vi "S4GUI.vi"() -> ()   [LabVIEW 2018] (continued)
            n2260 = call-dynamic "Write Observer.vi"("error in (no error)"=w5311, "Observer"=w5314, "Interface in"=w5310) -> ("error out"=w5306:errorcluster, "Interface out"=w5305:refnum<class "Interface.lvclass">)  [unwired: 7 in]
            n2261 = call-dynamic "Write Interface.vi"("error in (no error)"=w5306, "Interface.lvclass"=w5305, "Channel in"=w5325) -> ("error out"=w5301:errorcluster, "Channel out"=w5304:refnum<class "Channel.lvclass">)  [unwired: 7 in]
            n2262 = call-dynamic "Read State Machine.vi"("error in (no error)"=w5301, "Device in"=w5304) -> ("error out"=w5309:errorcluster, "State Machine.lvclass"=w5299:refnum<class "State Machine.lvclass">, "Device out"=w5303:refnum<class "Channel.lvclass">)  [unwired: 7 in]
            n2263 = call "Next State.vi"("error in (no error)"=w5309, "New_State"=12, "State Machine in"=w5299) -> ("error out"=w5308:errorcluster, "State Machine out"=w5298:refnum<class "State Machine.lvclass">)  [unwired: 7 in]
            n2264 = call-dynamic "Write State Machine.vi"("error in (no error)"=w5308, "State Machine.lvclass"=w5298, "Device in"=w5303) -> ("error out"=w5300:errorcluster, "Device out"=w5302:refnum<class "Channel.lvclass">)  [unwired: 7 in]
            n2265 = call-dynamic "Write Channel.vi"("error in (no error)"=w5300, "Channel.lvclass"=w5302, "Acquisition in"=w5320) -> ("error out"=w5318:errorcluster, "Acquisition out"=w5319:refnum<class "Acquisition.lvclass">)  [unwired: 7 in]
            n2266 = call-dynamic "Write AcquisitionD.vi"("error in (no error)"=w5318, "Acquisition.lvclass"=w5319, "S4ACS_GUI in"=w5321) -> ("error out"=w5332:errorcluster, "S4ACS_GUI out"=w5333:refnum<class "S4GUI.lvclass">)  [unwired: 7 in]
          }
        }
      }
      event "Start ch1": Value Change {
        n2267 = event-data() -> ()  [unwired: 1 in, 6 out]
        n2268 = call "Read Instrument.lvclass.vi"("error in (no error)"=w5341, "S4ACS_GUI in"=w5343) -> ("error out"=w5344:errorcluster, "Instrument.lvclass"=w5345:refnum<class "Instrument.lvclass">, "S4ACS_GUI out"=w5342:refnum<class "S4GUI.lvclass">)  [unwired: 7 in]
        n2269 = call-dynamic "Read mode.vi"("error in (no error)"=w5344, "Instrument in"=w5345) -> ("error out"=w5340:errorcluster, "mode"=w5339:bool)  [unwired: 7 in, 1 out]
        n2270 = call-dynamic "Read AcquisitionA.vi"("error in (no error)"=w5340, "S4ACS_GUI in"=w5342) -> ("error out"=w5357:errorcluster, "Acquisition.lvclass"=w5358:refnum<class "Acquisition.lvclass">, "S4ACS_GUI out"=w5360:refnum<class "S4GUI.lvclass">)  [unwired: 7 in]
        n2271 = call-dynamic "Read Acq_state.vi"("error in (no error)"=w5357, "Acquisition in"=w5358) -> ("error out"=w5354:errorcluster, "Acq_state"=w5356:u32, "Acquisition out"=w5353:refnum<class "Acquisition.lvclass">)  [unwired: 7 in]
        n2272 = Not Equal?(x=w5356, y=u32 400) -> (x != y?=w5359:bool)
        n2273 = case shown="True" w5359 {
          tunnel: w5360 -> [w5373 w5394]
          tunnel: [w5373 w5402] -> w5352
          tunnel: [w5361 w5400] -> w5336
          tunnel: w5354 -> [w5375 w5419]
          tunnel: w5353 -> [w5378 w5424]
          tunnel: [w5362 w5423] -> w5351
          tunnel: w5350 -> [_ w5421]
          tunnel: w5349 -> [_ w5420]
          tunnel: w5348 -> [_ w5418]
          tunnel: w5347 -> [_ w5417]
          tunnel: w5346 -> [_ w5412]
          tunnel: w5339 -> [_ w5399]
          frame False {
            n2274 = call-dynamic "Read Acq_prevstate.vi"("error in (no error)"=w5375, "Acquisition in"=w5378) -> ("error out"=w5374:errorcluster, "Acq_prevstate"=w5376:u32, "Acquisition out"=w5377:refnum<class "Acquisition.lvclass">)  [unwired: 7 in]
            n2275 = call-dynamic "Write Acq_state.vi"("error in (no error)"=w5374, "Acq_state"=w5376, "Acquisition in"=w5377) -> ("error out"=w5363:errorcluster, "Acquisition out"=w5364:refnum<class "Acquisition.lvclass">)  [unwired: 7 in]
            n2276 = call-dynamic "Read Channel.vi"("error in (no error)"=w5363, "Acquisition in"=w5364) -> ("error out"=w5367:errorcluster, "Channel.lvclass"=w5368:refnum<class "Channel.lvclass">, "Acquisition out"=w5372:refnum<class "Acquisition.lvclass">)  [unwired: 7 in]
            n2277 = call "Read connected.vi"("error in (no error)"=w5367, "Device in"=w5368) -> ("error out"=w5366:errorcluster, "connected"=w5365:bool, "Device out"=w5369:refnum<class "Channel.lvclass">)  [unwired: 7 in]
            n2278 = case shown="True" w5365 {
              tunnel: w5369 -> [w5380 w5390]
              tunnel: [w5380 w5388] -> w5371
              tunnel: w5366 -> [w5379 w5385]
              tunnel: [w5379 w5383] -> w5370
              frame False {
              }
              frame True {
                n2279 = call-dynamic "Read State Machine.vi"("error in (no error)"=w5385, "Device in"=w5390) -> ("error out"=w5381:errorcluster, "State Machine.lvclass"=w5382:refnum<class "State Machine.lvclass">, "Device out"=w5389:refnum<class "Channel.lvclass">)  [unwired: 7 in]
                n2280 = call "Next State.vi"("error in (no error)"=w5381, "New_State"=96, "State Machine in"=w5382) -> ("error out"=w5384:errorcluster, "State Machine out"=w5387:refnum<class "State Machine.lvclass">)  [unwired: 7 in]
                n2281 = call-dynamic "Write State Machine.vi"("error in (no error)"=w5384, "State Machine.lvclass"=w5387, "Device in"=w5389) -> ("error out"=w5383:errorcluster, "Device out"=w5388:refnum<class "Channel.lvclass">)  [unwired: 7 in]
              }
            }
            n2282 = call-dynamic "Write Channel.vi"("error in (no error)"=w5370, "Channel.lvclass"=w5371, "Acquisition in"=w5372) -> ("error out"=w5361:errorcluster, "Acquisition out"=w5362:refnum<class "Acquisition.lvclass">)  [unwired: 7 in]
          }
          frame True {
            # "object"
            # "suffix"
            # "obsType"
            n2283 = call "Read Instrument.lvclass.vi"("S4ACS_GUI in"=w5394) -> ("error out"=w5396:errorcluster, "Instrument.lvclass"=w5398:refnum<class "Instrument.lvclass">, "S4ACS_GUI out"=w5393:refnum<class "S4GUI.lvclass">)  [unwired: 8 in]
            n2284 = call "Read WPROT.vi"("error in (no error)"=w5396, "Instrument in"=w5398) -> ("error out"=w5395:errorcluster, "Opt_Selector.lvclass"=w5397:refnum<class "Opt_Selector.lvclass">)  [unwired: 7 in, 1 out]
            n2285 = call-dynamic "Read sequencia.vi"("error in (no error)"=w5395, "Opt_Selector in"=w5397) -> ("sequencia"=w5392:u16)  [unwired: 7 in, 2 out]
            n2286 = case shown="True" w5399 {
              tunnel: [0 w5459] -> w5391
              tunnel: w5392 -> [_ w5458]
              frame False {
                # "OV 20230424: \n#SEQ agora armazena as\nposições da lâmina utilizadas.\nNa fotometria, #SEQ=0"
                # "fotometria:"
              }
              frame True {
                # "OV 20230424: \n#SEQ agora armazena as\nposições da lâmina utilizadas.\nNa polarimetria, #SEQ=WPROT.sequencia"
                # "polarimetria:"
                n2287 = To Unsigned Long Integer(number=w5458) -> (unsigned 32bit integer=w5459:u32)
              }
            }
            n2288 = call-dynamic "Write Acq_state.vi"("error in (no error)"=w5419, "Acq_state"=u32 251, "Acquisition in"=w5424) -> ("error out"=w5425:errorcluster, "Acquisition out"=w5426:refnum<class "Acquisition.lvclass">)  [unwired: 7 in]
            n2289 = call-dynamic "Read Channel.vi"("error in (no error)"=w5425, "Acquisition in"=w5426) -> ("error out"=w5428:errorcluster, "Channel.lvclass"=w5429:refnum<class "Channel.lvclass">, "Acquisition out"=w5441:refnum<class "Acquisition.lvclass">)  [unwired: 7 in]
            n2290 = property on="Start ch1" class="Bool"(error in=w5419, "DisabledEnum"=T7."Disabled and Grayed Out" ("Disabled")) -> ()  [unwired: 1 in, 2 out]
            n2291 = call-dynamic "Read Interface.vi"("error in (no error)"=w5428, "Channel in"=w5429) -> ("error out"=w5455:errorcluster, "Interface.lvclass"=w5456:refnum<class "Interface.lvclass">, "Channel out"=w5454:refnum<class "Channel.lvclass">)  [unwired: 7 in]
            n2292 = call "Write Exposure Time.vi"("error in (no error)"=w5455, "Exposure Time"="Exptime ch1", "Interface in"=w5456) -> ("error out"=w5452:errorcluster, "Interface out"=w5453:refnum<class "Interface.lvclass">)  [unwired: 7 in]
            n2293 = call-dynamic "Write # Index.vi"("error in (no error)"=w5452, "# Index"="Index ch1", "Interface in"=w5453) -> ("error out"=w5450:errorcluster, "Interface out"=w5451:refnum<class "Interface.lvclass">)  [unwired: 7 in]
            n2294 = call-dynamic "Write Suffix.vi"("error in (no error)"=w5450, "Suffix"=w5421, "Interface in"=w5451) -> ("error out"=w5449:errorcluster, "Interface out"=w5448:refnum<class "Interface.lvclass">)  [unwired: 7 in]
            n2295 = call-dynamic "Write ObsType.vi"("error in (no error)"=w5449, "ObsType"=w5418, "Interface in"=w5448) -> ("error out"=w5446:errorcluster, "Interface out"=w5447:refnum<class "Interface.lvclass">)  [unwired: 7 in]
            n2296 = call-dynamic "Write Object.vi"("error in (no error)"=w5446, "Object"=w5417, "Interface in"=w5447) -> ("error out"=w5445:errorcluster, "Interface out"=w5444:refnum<class "Interface.lvclass">)  [unwired: 7 in]
            n2297 = call-dynamic "Write Comments.vi"("error in (no error)"=w5445, "Comments"=w5420, "Interface in"=w5444) -> ("error out"=w5442:errorcluster, "Interface out"=w5443:refnum<class "Interface.lvclass">)  [unwired: 7 in]
            n2298 = call-dynamic "Write DS9.vi"("error in (no error)"=w5442, "DS9"="F", "Interface in"=w5443) -> ("error out"=w5414:errorcluster, "Interface out"=w5416:refnum<class "Interface.lvclass">)  [unwired: 7 in]
            n2299 = call-dynamic "Write Observer.vi"("error in (no error)"=w5414, "Observer"=w5412, "Interface in"=w5416) -> ("error out"=w5413:errorcluster, "Interface out"=w5415:refnum<class "Interface.lvclass">)  [unwired: 7 in]
            n2300 = call-dynamic "Write # Images.vi"("error in (no error)"=w5413, "# Images"="Exp ch1", "Interface in"=w5415) -> ("error out"=w5437:errorcluster, "Interface out"=w5440:refnum<class "Interface.lvclass">)  [unwired: 7 in]
            n2301 = call-dynamic "Write Interface.vi"("error in (no error)"=w5437, "Interface.lvclass"=w5440, "Channel in"=w5454) -> ("error out"=w5430:errorcluster, "Channel out"=w5431:refnum<class "Channel.lvclass">)  [unwired: 7 in]
            n2302 = property on="Exposure Time ch1" class="Slide (strict)"("Scale.Maximum"="Exptime ch1", "Scale.Minimum"=0.0 ("Scale.Range:Minimum")) -> ()  [unwired: 2 in, 2 out]
            n2303 = property on="Cycles Done ch1" class="Slide (strict)"("Scale.Maximum"="#cycles ch1", "Scale.Minimum"=0.0 ("Scale.Range:Minimum")) -> ()  [unwired: 2 in, 2 out]
            n2304 = property on="Exposure Done ch1" class="Slide (strict)"("Scale.Maximum"="Exp ch1", "Scale.Minimum"=0.0 ("Scale.Range:Minimum")) -> ()  [unwired: 2 in, 2 out]
            n2305 = call-dynamic "Write ciclos.vi"("error in (no error)"=w5430, "ciclos"="#cycles ch1", "Channel in"=w5431) -> ("error out"=w5410:errorcluster, "Channel out"=w5411:refnum<class "Channel.lvclass">)  [unwired: 7 in]
            n2306 = call-dynamic "Write sequencias.vi"("error in (no error)"=w5410, "sequencias"=w5391, "Channel in"=w5411) -> ("error out"=w5409:errorcluster, "Channel out"=w5408:refnum<class "Channel.lvclass">)  [unwired: 7 in]
            n2307 = call-dynamic "Write Channel.vi"("error in (no error)"=w5409, "Channel.lvclass"=w5408, "Acquisition in"=w5441) -> ("error out"=w5401:errorcluster, "Acquisition out"=w5423:refnum<class "Acquisition.lvclass">)  [unwired: 7 in]
            n2308 = call-dynamic "Write sequencias.vi"("error in (no error)"=w5401, "sequencias"=w5391, "S4GUI in"=w5393) -> ("error out"=w5405:errorcluster, "S4GUI out"=w5404:refnum<class "S4GUI.lvclass">)  [unwired: 7 in]
            n2309 = call-dynamic "Write ciclos.vi"("error in (no error)"=w5405, "ciclos"="#cycles ch1", "S4ACS_GUI in"=w5404) -> ("error out"=w5406:errorcluster, "S4ACS_GUI out"=w5407:refnum<class "S4GUI.lvclass">)  [unwired: 7 in]
            n2310 = call-dynamic "Write TotalCiclos.vi"("error in (no error)"=w5406, "TotalCiclos"="#cycles ch1", "S4GUI in"=w5407) -> ("error out"=w5400:errorcluster, "S4GUI out"=w5402:refnum<class "S4GUI.lvclass">)  [unwired: 7 in]
          }
        }
        n2311 = call-dynamic "Write AcquisitionA.vi"("error in (no error)"=w5336, "Acquisition.lvclass"=w5351, "S4ACS_GUI in"=w5352) -> ("error out"=w5337:errorcluster, "S4ACS_GUI out"=w5338:refnum<class "S4GUI.lvclass">)  [unwired: 7 in]
      }
      event "Start ch2": Value Change {
        n2312 = event-data() -> ()  [unwired: 1 in, 6 out]
        n2313 = call "Read Instrument.lvclass.vi"("error in (no error)"=w5464, "S4ACS_GUI in"=w5465) -> ("error out"=w5466:errorcluster, "Instrument.lvclass"=w5467:refnum<class "Instrument.lvclass">, "S4ACS_GUI out"=w5463:refnum<class "S4GUI.lvclass">)  [unwired: 7 in]
        n2314 = call-dynamic "Read mode.vi"("error in (no error)"=w5466, "Instrument in"=w5467) -> ("error out"=w5462:errorcluster, "mode"=w5461:bool)  [unwired: 7 in, 1 out]
        n2315 = call "Read AcquisitionB.vi"("error in (no error)"=w5462, "S4ACS_GUI in"=w5463) -> ("error out"=w5481:errorcluster, "Acquisition.lvclass"=w5482:refnum<class "Acquisition.lvclass">, "S4ACS_GUI out"=w5484:refnum<class "S4GUI.lvclass">)  [unwired: 7 in]
        n2316 = call-dynamic "Read Acq_state.vi"("error in (no error)"=w5481, "Acquisition in"=w5482) -> ("error out"=w5478:errorcluster, "Acq_state"=w5480:u32, "Acquisition out"=w5477:refnum<class "Acquisition.lvclass">)  [unwired: 7 in]
        n2317 = Not Equal?(x=w5480, y=u32 400) -> (x != y?=w5483:bool)
        n2318 = case shown="True" w5483 {
          tunnel: w5484 -> [w5497 w5519]
          tunnel: [w5497 w5527] -> w5476
          tunnel: [w5485 w5525] -> w5460
          tunnel: w5478 -> [w5499 w5547]
          tunnel: w5477 -> [w5502 w5553]
          tunnel: [w5486 w5552] -> w5475
          tunnel: w5473 -> [_ w5549]
          tunnel: w5472 -> [_ w5548]
          tunnel: w5470 -> [_ w5543]
          tunnel: w5469 -> [_ w5542]
          tunnel: w5468 -> [_ w5536]
          tunnel: w5461 -> [_ w5516]
          frame False {
            n2319 = call-dynamic "Read Acq_prevstate.vi"("error in (no error)"=w5499, "Acquisition in"=w5502) -> ("error out"=w5498:errorcluster, "Acq_prevstate"=w5500:u32, "Acquisition out"=w5501:refnum<class "Acquisition.lvclass">)  [unwired: 7 in]
            n2320 = call-dynamic "Write Acq_state.vi"("error in (no error)"=w5498, "Acq_state"=w5500, "Acquisition in"=w5501) -> ("error out"=w5487:errorcluster, "Acquisition out"=w5488:refnum<class "Acquisition.lvclass">)  [unwired: 7 in]
            n2321 = call-dynamic "Read Channel.vi"("error in (no error)"=w5487, "Acquisition in"=w5488) -> ("error out"=w5491:errorcluster, "Channel.lvclass"=w5492:refnum<class "Channel.lvclass">, "Acquisition out"=w5496:refnum<class "Acquisition.lvclass">)  [unwired: 7 in]
            n2322 = call "Read connected.vi"("error in (no error)"=w5491, "Device in"=w5492) -> ("error out"=w5490:errorcluster, "connected"=w5489:bool, "Device out"=w5493:refnum<class "Channel.lvclass">)  [unwired: 7 in]
            n2323 = case shown="True" w5489 {
              tunnel: w5493 -> [w5504 w5514]
              tunnel: [w5504 w5512] -> w5495
              tunnel: w5490 -> [w5503 w5509]
              tunnel: [w5503 w5507] -> w5494
              frame False {
              }
              frame True {
                n2324 = call-dynamic "Read State Machine.vi"("error in (no error)"=w5509, "Device in"=w5514) -> ("error out"=w5505:errorcluster, "State Machine.lvclass"=w5506:refnum<class "State Machine.lvclass">, "Device out"=w5513:refnum<class "Channel.lvclass">)  [unwired: 7 in]
                n2325 = call "Next State.vi"("error in (no error)"=w5505, "New_State"=96, "State Machine in"=w5506) -> ("error out"=w5508:errorcluster, "State Machine out"=w5511:refnum<class "State Machine.lvclass">)  [unwired: 7 in]
                n2326 = call-dynamic "Write State Machine.vi"("error in (no error)"=w5508, "State Machine.lvclass"=w5511, "Device in"=w5513) -> ("error out"=w5507:errorcluster, "Device out"=w5512:refnum<class "Channel.lvclass">)  [unwired: 7 in]
              }
            }
            n2327 = call-dynamic "Write Channel.vi"("error in (no error)"=w5494, "Channel.lvclass"=w5495, "Acquisition in"=w5496) -> ("error out"=w5485:errorcluster, "Acquisition out"=w5486:refnum<class "Acquisition.lvclass">)  [unwired: 7 in]
          }
          frame True {
            # "obs type"
            # "suffix"
            # "object"
            n2328 = call "Read Instrument.lvclass.vi"("S4ACS_GUI in"=w5519) -> ("error out"=w5521:errorcluster, "Instrument.lvclass"=w5523:refnum<class "Instrument.lvclass">, "S4ACS_GUI out"=w5518:refnum<class "S4GUI.lvclass">)  [unwired: 8 in]
            n2329 = call "Read WPROT.vi"("error in (no error)"=w5521, "Instrument in"=w5523) -> ("error out"=w5520:errorcluster, "Opt_Selector.lvclass"=w5522:refnum<class "Opt_Selector.lvclass">)  [unwired: 7 in, 1 out]
            n2330 = call-dynamic "Read sequencia.vi"("error in (no error)"=w5520, "Opt_Selector in"=w5522) -> ("sequencia"=w5515:u16)  [unwired: 7 in, 2 out]
            n2331 = case shown="True" w5516 {
              tunnel: [0 w5583] -> w5517
              tunnel: w5515 -> [_ w5582]
              frame False {
                # "OV 20230424: \n#SEQ agora armazena as\nposições da lâmina utilizadas.\nNa fotometria, #SEQ=0"
                # "fotometria:"
              }
              frame True {
                # "OV 20230424: \n#SEQ agora armazena as\nposições da lâmina utilizadas.\nNa polarimetria, #SEQ=WPROT.sequencia"
                # "polarimetria:"
                n2332 = To Unsigned Long Integer(number=w5582) -> (unsigned 32bit integer=w5583:u32)
              }
            }
            n2333 = call-dynamic "Write Acq_state.vi"("error in (no error)"=w5547, "Acq_state"=u32 251, "Acquisition in"=w5553) -> ("error out"=w5554:errorcluster, "Acquisition out"=w5555:refnum<class "Acquisition.lvclass">)  [unwired: 7 in]
            n2334 = call-dynamic "Read Channel.vi"("error in (no error)"=w5554, "Acquisition in"=w5555) -> ("error out"=w5557:errorcluster, "Channel.lvclass"=w5558:refnum<class "Channel.lvclass">, "Acquisition out"=w5565:refnum<class "Acquisition.lvclass">)  [unwired: 7 in]
            n2335 = property on="Start ch2" class="Bool"(error in=w5547, "DisabledEnum"=T7."Disabled and Grayed Out" ("Disabled")) -> ()  [unwired: 1 in, 2 out]
            n2336 = call-dynamic "Read Interface.vi"("error in (no error)"=w5557, "Channel in"=w5558) -> ("error out"=w5579:errorcluster, "Interface.lvclass"=w5580:refnum<class "Interface.lvclass">, "Channel out"=w5578:refnum<class "Channel.lvclass">)  [unwired: 7 in]
            n2337 = call "Write Exposure Time.vi"("error in (no error)"=w5579, "Exposure Time"="Exptime ch2", "Interface in"=w5580) -> ("error out"=w5576:errorcluster, "Interface out"=w5577:refnum<class "Interface.lvclass">)  [unwired: 7 in]
            n2338 = call-dynamic "Write # Index.vi"("error in (no error)"=w5576, "# Index"="Index ch2", "Interface in"=w5577) -> ("error out"=w5574:errorcluster, "Interface out"=w5575:refnum<class "Interface.lvclass">)  [unwired: 7 in]
            n2339 = call-dynamic "Write Suffix.vi"("error in (no error)"=w5574, "Suffix"=w5549, "Interface in"=w5575) -> ("error out"=w5573:errorcluster, "Interface out"=w5572:refnum<class "Interface.lvclass">)  [unwired: 7 in]
            n2340 = call-dynamic "Write ObsType.vi"("error in (no error)"=w5573, "ObsType"=w5543, "Interface in"=w5572) -> ("error out"=w5570:errorcluster, "Interface out"=w5571:refnum<class "Interface.lvclass">)  [unwired: 7 in]
            n2341 = call-dynamic "Write Object.vi"("error in (no error)"=w5570, "Object"=w5542, "Interface in"=w5571) -> ("error out"=w5569:errorcluster, "Interface out"=w5568:refnum<class "Interface.lvclass">)  [unwired: 7 in]
            n2342 = call-dynamic "Write Comments.vi"("error in (no error)"=w5569, "Comments"=w5548, "Interface in"=w5568) -> ("error out"=w5566:errorcluster, "Interface out"=w5567:refnum<class "Interface.lvclass">)  [unwired: 7 in]
            n2343 = call-dynamic "Write DS9.vi"("error in (no error)"=w5566, "DS9"="F", "Interface in"=w5567) -> ("error out"=w5539:errorcluster, "Interface out"=w5541:refnum<class "Interface.lvclass">)  [unwired: 7 in]
            n2344 = call-dynamic "Write Observer.vi"("error in (no error)"=w5539, "Observer"=w5536, "Interface in"=w5541) -> ("error out"=w5538:errorcluster, "Interface out"=w5540:refnum<class "Interface.lvclass">)  [unwired: 7 in]
            n2345 = call-dynamic "Write # Images.vi"("error in (no error)"=w5538, "# Images"="Exp ch2", "Interface in"=w5540) -> ("error out"=w5545:errorcluster, "Interface out"=w5544:refnum<class "Interface.lvclass">)  [unwired: 7 in]
            n2346 = property on="Exposure Time ch2" class="Slide (strict)"("Scale.Maximum"="Exptime ch2", "Scale.Minimum"=0.0 ("Scale.Range:Minimum")) -> ()  [unwired: 2 in, 2 out]
            n2347 = property on="Cycles Done ch2" class="Slide (strict)"("Scale.Maximum"="#cycles ch2", "Scale.Minimum"=0.0 ("Scale.Range:Minimum")) -> ()  [unwired: 2 in, 2 out]
            n2348 = property on="Exposure Done ch2" class="Slide (strict)"("Scale.Maximum"="Exp ch2", "Scale.Minimum"=0.0 ("Scale.Range:Minimum")) -> ()  [unwired: 2 in, 2 out]
            n2349 = call-dynamic "Write Interface.vi"("error in (no error)"=w5545, "Interface.lvclass"=w5544, "Channel in"=w5578) -> ("error out"=w5559:errorcluster, "Channel out"=w5560:refnum<class "Channel.lvclass">)  [unwired: 7 in]
            n2350 = call-dynamic "Write ciclos.vi"("error in (no error)"=w5559, "ciclos"="#cycles ch2", "Channel in"=w5560) -> ("error out"=w5535:errorcluster, "Channel out"=w5534:refnum<class "Channel.lvclass">)  [unwired: 7 in]
            n2351 = call-dynamic "Write sequencias.vi"("error in (no error)"=w5535, "sequencias"=w5517, "Channel in"=w5534) -> ("error out"=w5533:errorcluster, "Channel out"=w5532:refnum<class "Channel.lvclass">)  [unwired: 7 in]
            n2352 = call-dynamic "Write Channel.vi"("error in (no error)"=w5533, "Channel.lvclass"=w5532, "Acquisition in"=w5565) -> ("error out"=w5526:errorcluster, "Acquisition out"=w5552:refnum<class "Acquisition.lvclass">)  [unwired: 7 in]
            n2353 = call-dynamic "Write sequencias.vi"("error in (no error)"=w5526, "sequencias"=w5517, "S4GUI in"=w5518) -> ("error out"=w5529:errorcluster, "S4GUI out"=w5528:refnum<class "S4GUI.lvclass">)  [unwired: 7 in]
            n2354 = call-dynamic "Write ciclos.vi"("error in (no error)"=w5529, "ciclos"="#cycles ch2", "S4ACS_GUI in"=w5528) -> ("error out"=w5530:errorcluster, "S4ACS_GUI out"=w5531:refnum<class "S4GUI.lvclass">)  [unwired: 7 in]
            n2355 = call-dynamic "Write TotalCiclos.vi"("error in (no error)"=w5530, "TotalCiclos"="#cycles ch2", "S4GUI in"=w5531) -> ("error out"=w5525:errorcluster, "S4GUI out"=w5527:refnum<class "S4GUI.lvclass">)  [unwired: 7 in]
          }
        }
        n2356 = call "Write AcquisitionB.vi"("error in (no error)"=w5460, "Acquisition.lvclass"=w5475, "S4ACS_GUI in"=w5476) -> ("error out"=w5474:errorcluster, "S4ACS_GUI out"=w5471:refnum<class "S4GUI.lvclass">)  [unwired: 7 in]
      }
      event "Start ch3": Value Change {
        n2357 = event-data() -> ()  [unwired: 1 in, 6 out]
        n2358 = call "Read Instrument.lvclass.vi"("error in (no error)"=w5587, "S4ACS_GUI in"=w5589) -> ("error out"=w5590:errorcluster, "Instrument.lvclass"=w5591:refnum<class "Instrument.lvclass">, "S4ACS_GUI out"=w5588:refnum<class "S4GUI.lvclass">)  [unwired: 7 in]
        n2359 = call-dynamic "Read mode.vi"("error in (no error)"=w5590, "Instrument in"=w5591) -> ("error out"=w5586:errorcluster, "mode"=w5585:bool)  [unwired: 7 in, 1 out]
        n2360 = call-dynamic "Read AcquisitionC.vi"("error in (no error)"=w5586, "S4ACS_GUI in"=w5588) -> ("error out"=w5605:errorcluster, "Acquisition.lvclass"=w5606:refnum<class "Acquisition.lvclass">, "S4ACS_GUI out"=w5608:refnum<class "S4GUI.lvclass">)  [unwired: 7 in]
        n2361 = call-dynamic "Read Acq_state.vi"("error in (no error)"=w5605, "Acquisition in"=w5606) -> ("error out"=w5602:errorcluster, "Acq_state"=w5604:u32, "Acquisition out"=w5601:refnum<class "Acquisition.lvclass">)  [unwired: 7 in]
        n2362 = Not Equal?(x=w5604, y=u32 400) -> (x != y?=w5607:bool)
        n2363 = case shown="True" w5607 {
          tunnel: w5608 -> [w5621 w5641]
          tunnel: [w5621 w5649] -> w5600
          tunnel: [w5609 w5650] -> w5584
          tunnel: w5602 -> [w5623 w5670]
          tunnel: w5601 -> [w5626 w5676]
          tunnel: [w5610 w5675] -> w5599
          tunnel: w5597 -> [_ w5672]
          tunnel: w5596 -> [_ w5671]
          tunnel: w5594 -> [_ w5666]
          tunnel: w5593 -> [_ w5665]
          tunnel: w5592 -> [_ w5660]
          tunnel: w5585 -> [_ w5646]
          frame False {
            n2364 = call-dynamic "Read Acq_prevstate.vi"("error in (no error)"=w5623, "Acquisition in"=w5626) -> ("error out"=w5622:errorcluster, "Acq_prevstate"=w5624:u32, "Acquisition out"=w5625:refnum<class "Acquisition.lvclass">)  [unwired: 7 in]
            n2365 = call-dynamic "Write Acq_state.vi"("error in (no error)"=w5622, "Acq_state"=w5624, "Acquisition in"=w5625) -> ("error out"=w5614:errorcluster, "Acquisition out"=w5615:refnum<class "Acquisition.lvclass">)  [unwired: 7 in]
            n2366 = call-dynamic "Read Channel.vi"("error in (no error)"=w5614, "Acquisition in"=w5615) -> ("error out"=w5618:errorcluster, "Channel.lvclass"=w5612:refnum<class "Channel.lvclass">, "Acquisition out"=w5613:refnum<class "Acquisition.lvclass">)  [unwired: 7 in]
            n2367 = call "Read connected.vi"("error in (no error)"=w5618, "Device in"=w5612) -> ("error out"=w5617:errorcluster, "connected"=w5616:bool, "Device out"=w5619:refnum<class "Channel.lvclass">)  [unwired: 7 in]
            n2368 = case shown="True" w5616 {
              tunnel: w5619 -> [w5628 w5638]
              tunnel: [w5628 w5636] -> w5611
              tunnel: w5617 -> [w5627 w5633]
              tunnel: [w5627 w5631] -> w5620
              frame False {
              }
              frame True {
                n2369 = call-dynamic "Read State Machine.vi"("error in (no error)"=w5633, "Device in"=w5638) -> ("error out"=w5629:errorcluster, "State Machine.lvclass"=w5630:refnum<class "State Machine.lvclass">, "Device out"=w5637:refnum<class "Channel.lvclass">)  [unwired: 7 in]
                n2370 = call "Next State.vi"("error in (no error)"=w5629, "New_State"=96, "State Machine in"=w5630) -> ("error out"=w5632:errorcluster, "State Machine out"=w5635:refnum<class "State Machine.lvclass">)  [unwired: 7 in]
                n2371 = call-dynamic "Write State Machine.vi"("error in (no error)"=w5632, "State Machine.lvclass"=w5635, "Device in"=w5637) -> ("error out"=w5631:errorcluster, "Device out"=w5636:refnum<class "Channel.lvclass">)  [unwired: 7 in]
              }
            }
            n2372 = call-dynamic "Write Channel.vi"("error in (no error)"=w5620, "Channel.lvclass"=w5611, "Acquisition in"=w5613) -> ("error out"=w5609:errorcluster, "Acquisition out"=w5610:refnum<class "Acquisition.lvclass">)  [unwired: 7 in]
          }
          frame True {
            # "obs type"
            # "suffix"
            # "object"
            n2373 = call "Read Instrument.lvclass.vi"("S4ACS_GUI in"=w5641) -> ("error out"=w5643:errorcluster, "Instrument.lvclass"=w5645:refnum<class "Instrument.lvclass">, "S4ACS_GUI out"=w5640:refnum<class "S4GUI.lvclass">)  [unwired: 8 in]
            n2374 = call "Read WPROT.vi"("error in (no error)"=w5643, "Instrument in"=w5645) -> ("error out"=w5642:errorcluster, "Opt_Selector.lvclass"=w5644:refnum<class "Opt_Selector.lvclass">)  [unwired: 7 in, 1 out]
            n2375 = call-dynamic "Read sequencia.vi"("error in (no error)"=w5642, "Opt_Selector in"=w5644) -> ("sequencia"=w5639:u16)  [unwired: 7 in, 2 out]
            n2376 = case shown="True" w5646 {
              tunnel: [0 w5707] -> w5647
              tunnel: w5639 -> [_ w5706]
              frame False {
                # "OV 20230424: \n#SEQ agora armazena as\nposições da lâmina utilizadas.\nNa fotometria, #SEQ=0"
                # "fotometria:"
              }
              frame True {
                # "OV 20230424: \n#SEQ agora armazena as\nposições da lâmina utilizadas.\nNa polarimetria, #SEQ=WPROT.sequencia"
                # "polarimetria:"
                n2377 = To Unsigned Long Integer(number=w5706) -> (unsigned 32bit integer=w5707:u32)
              }
            }
            n2378 = call-dynamic "Write Acq_state.vi"("error in (no error)"=w5670, "Acq_state"=u32 251, "Acquisition in"=w5676) -> ("error out"=w5677:errorcluster, "Acquisition out"=w5678:refnum<class "Acquisition.lvclass">)  [unwired: 7 in]
            n2379 = call-dynamic "Read Channel.vi"("error in (no error)"=w5677, "Acquisition in"=w5678) -> ("error out"=w5680:errorcluster, "Channel.lvclass"=w5681:refnum<class "Channel.lvclass">, "Acquisition out"=w5689:refnum<class "Acquisition.lvclass">)  [unwired: 7 in]
            n2380 = property on="Start ch3" class="Bool"(error in=w5670, "DisabledEnum"=T7."Disabled and Grayed Out" ("Disabled")) -> ()  [unwired: 1 in, 2 out]
            n2381 = call-dynamic "Read Interface.vi"("error in (no error)"=w5680, "Channel in"=w5681) -> ("error out"=w5703:errorcluster, "Interface.lvclass"=w5704:refnum<class "Interface.lvclass">, "Channel out"=w5702:refnum<class "Channel.lvclass">)  [unwired: 7 in]
            n2382 = call "Write Exposure Time.vi"("error in (no error)"=w5703, "Exposure Time"="Exptime ch3", "Interface in"=w5704) -> ("error out"=w5700:errorcluster, "Interface out"=w5701:refnum<class "Interface.lvclass">)  [unwired: 7 in]
            n2383 = call-dynamic "Write # Index.vi"("error in (no error)"=w5700, "# Index"="Index ch3", "Interface in"=w5701) -> ("error out"=w5698:errorcluster, "Interface out"=w5699:refnum<class "Interface.lvclass">)  [unwired: 7 in]
            n2384 = call-dynamic "Write Suffix.vi"("error in (no error)"=w5698, "Suffix"=w5672, "Interface in"=w5699) -> ("error out"=w5697:errorcluster, "Interface out"=w5696:refnum<class "Interface.lvclass">)  [unwired: 7 in]
            n2385 = call-dynamic "Write ObsType.vi"("error in (no error)"=w5697, "ObsType"=w5665, "Interface in"=w5696) -> ("error out"=w5694:errorcluster, "Interface out"=w5695:refnum<class "Interface.lvclass">)  [unwired: 7 in]
            n2386 = call-dynamic "Write Object.vi"("error in (no error)"=w5694, "Object"=w5666, "Interface in"=w5695) -> ("error out"=w5693:errorcluster, "Interface out"=w5692:refnum<class "Interface.lvclass">)  [unwired: 7 in]
            n2387 = call-dynamic "Write Comments.vi"("error in (no error)"=w5693, "Comments"=w5671, "Interface in"=w5692) -> ("error out"=w5690:errorcluster, "Interface out"=w5691:refnum<class "Interface.lvclass">)  [unwired: 7 in]
            n2388 = call-dynamic "Write DS9.vi"("error in (no error)"=w5690, "DS9"="F", "Interface in"=w5691) -> ("error out"=w5662:errorcluster, "Interface out"=w5664:refnum<class "Interface.lvclass">)  [unwired: 7 in]
            n2389 = call-dynamic "Write Observer.vi"("error in (no error)"=w5662, "Observer"=w5660, "Interface in"=w5664) -> ("error out"=w5661:errorcluster, "Interface out"=w5663:refnum<class "Interface.lvclass">)  [unwired: 7 in]
            n2390 = call-dynamic "Write # Images.vi"("error in (no error)"=w5661, "# Images"="Exp ch3", "Interface in"=w5663) -> ("error out"=w5667:errorcluster, "Interface out"=w5668:refnum<class "Interface.lvclass">)  [unwired: 7 in]
            n2391 = property on="Exposure Time ch3" class="Slide (strict)"("Scale.Maximum"="Exptime ch3", "Scale.Minimum"=0.0 ("Scale.Range:Minimum")) -> ()  [unwired: 2 in, 2 out]
            n2392 = property on="Exposure Done ch3" class="Slide (strict)"("Scale.Maximum"="Exp ch3", "Scale.Minimum"=0.0 ("Scale.Range:Minimum")) -> ()  [unwired: 2 in, 2 out]
            n2393 = property on="Cycles Done ch3" class="Slide (strict)"("Scale.Maximum"="#cycles ch3", "Scale.Minimum"=0.0 ("Scale.Range:Minimum")) -> ()  [unwired: 2 in, 2 out]
            n2394 = call-dynamic "Write Interface.vi"("error in (no error)"=w5667, "Interface.lvclass"=w5668, "Channel in"=w5702) -> ("error out"=w5682:errorcluster, "Channel out"=w5683:refnum<class "Channel.lvclass">)  [unwired: 7 in]
            n2395 = call-dynamic "Write ciclos.vi"("error in (no error)"=w5682, "ciclos"="#cycles ch3", "Channel in"=w5683) -> ("error out"=w5658:errorcluster, "Channel out"=w5659:refnum<class "Channel.lvclass">)  [unwired: 7 in]
            n2396 = call-dynamic "Write sequencias.vi"("error in (no error)"=w5658, "sequencias"=w5647, "Channel in"=w5659) -> ("error out"=w5656:errorcluster, "Channel out"=w5657:refnum<class "Channel.lvclass">)  [unwired: 7 in]
            n2397 = call-dynamic "Write Channel.vi"("error in (no error)"=w5656, "Channel.lvclass"=w5657, "Acquisition in"=w5689) -> ("error out"=w5651:errorcluster, "Acquisition out"=w5675:refnum<class "Acquisition.lvclass">)  [unwired: 7 in]
            n2398 = call-dynamic "Write sequencias.vi"("error in (no error)"=w5651, "sequencias"=w5647, "S4GUI in"=w5640) -> ("error out"=w5653:errorcluster, "S4GUI out"=w5652:refnum<class "S4GUI.lvclass">)  [unwired: 7 in]
            n2399 = call-dynamic "Write ciclos.vi"("error in (no error)"=w5653, "ciclos"="#cycles ch3", "S4ACS_GUI in"=w5652) -> ("error out"=w5654:errorcluster, "S4ACS_GUI out"=w5655:refnum<class "S4GUI.lvclass">)  [unwired: 7 in]
            n2400 = call-dynamic "Write TotalCiclos.vi"("error in (no error)"=w5654, "TotalCiclos"="#cycles ch3", "S4GUI in"=w5655) -> ("error out"=w5650:errorcluster, "S4GUI out"=w5649:refnum<class "S4GUI.lvclass">)  [unwired: 7 in]
          }
        }
        n2401 = call-dynamic "Write AcquisitionC.vi"("error in (no error)"=w5584, "Acquisition.lvclass"=w5599, "S4ACS_GUI in"=w5600) -> ("error out"=w5598:errorcluster, "S4ACS_GUI out"=w5595:refnum<class "S4GUI.lvclass">)  [unwired: 7 in]
      }
      event "Start ch4": Value Change {
        n2402 = event-data() -> ()  [unwired: 1 in, 6 out]
        n2403 = call "Read Instrument.lvclass.vi"("error in (no error)"=w5713, "S4ACS_GUI in"=w5714) -> ("error out"=w5715:errorcluster, "Instrument.lvclass"=w5716:refnum<class "Instrument.lvclass">, "S4ACS_GUI out"=w5712:refnum<class "S4GUI.lvclass">)  [unwired: 7 in]
        n2404 = call-dynamic "Read mode.vi"("error in (no error)"=w5715, "Instrument in"=w5716) -> ("error out"=w5711:errorcluster, "mode"=w5710:bool)  [unwired: 7 in, 1 out]
        n2405 = call-dynamic "Read AcquisitionD.vi"("error in (no error)"=w5711, "S4ACS_GUI in"=w5712) -> ("error out"=w5729:errorcluster, "Acquisition.lvclass"=w5730:refnum<class "Acquisition.lvclass">, "S4ACS_GUI out"=w5732:refnum<class "S4GUI.lvclass">)  [unwired: 7 in]
        n2406 = call-dynamic "Read Acq_state.vi"("error in (no error)"=w5729, "Acquisition in"=w5730) -> ("error out"=w5726:errorcluster, "Acq_state"=w5728:u32, "Acquisition out"=w5725:refnum<class "Acquisition.lvclass">)  [unwired: 7 in]
        n2407 = Not Equal?(x=w5728, y=u32 400) -> (x != y?=w5731:bool)
        n2408 = case shown="True" w5731 {
          tunnel: w5732 -> [w5745 w5765]
          tunnel: [w5734 w5773] -> w5709
          tunnel: w5726 -> [w5747 w5794]
          tunnel: w5725 -> [w5750 w5800]
          tunnel: [w5733 w5799] -> w5724
          tunnel: w5722 -> [_ w5796]
          tunnel: w5721 -> [_ w5795]
          tunnel: w5719 -> [_ w5790]
          tunnel: w5718 -> [_ w5789]
          tunnel: w5717 -> [_ w5784]
          tunnel: w5710 -> [_ w5771]
          tunnel: [w5745 w5775] -> w5708
          frame False {
            n2409 = call-dynamic "Read Acq_prevstate.vi"("error in (no error)"=w5747, "Acquisition in"=w5750) -> ("error out"=w5746:errorcluster, "Acq_prevstate"=w5748:u32, "Acquisition out"=w5749:refnum<class "Acquisition.lvclass">)  [unwired: 7 in]
            n2410 = call-dynamic "Write Acq_state.vi"("error in (no error)"=w5746, "Acq_state"=w5748, "Acquisition in"=w5749) -> ("error out"=w5735:errorcluster, "Acquisition out"=w5736:refnum<class "Acquisition.lvclass">)  [unwired: 7 in]
            n2411 = call-dynamic "Read Channel.vi"("error in (no error)"=w5735, "Acquisition in"=w5736) -> ("error out"=w5742:errorcluster, "Channel.lvclass"=w5738:refnum<class "Channel.lvclass">, "Acquisition out"=w5739:refnum<class "Acquisition.lvclass">)  [unwired: 7 in]
            n2412 = call "Read connected.vi"("error in (no error)"=w5742, "Device in"=w5738) -> ("error out"=w5741:errorcluster, "connected"=w5740:bool, "Device out"=w5743:refnum<class "Channel.lvclass">)  [unwired: 7 in]
            n2413 = case shown="True" w5740 {
              tunnel: w5743 -> [w5752 w5762]
              tunnel: [w5752 w5760] -> w5737
              tunnel: w5741 -> [w5751 w5757]
              tunnel: [w5751 w5755] -> w5744
              frame False {
              }
              frame True {
                n2414 = call-dynamic "Read State Machine.vi"("error in (no error)"=w5757, "Device in"=w5762) -> ("error out"=w5753:errorcluster, "State Machine.lvclass"=w5754:refnum<class "State Machine.lvclass">, "Device out"=w5761:refnum<class "Channel.lvclass">)  [unwired: 7 in]
                n2415 = call "Next State.vi"("error in (no error)"=w5753, "New_State"=96, "State Machine in"=w5754) -> ("error out"=w5756:errorcluster, "State Machine out"=w5759:refnum<class "State Machine.lvclass">)  [unwired: 7 in]
                n2416 = call-dynamic "Write State Machine.vi"("error in (no error)"=w5756, "State Machine.lvclass"=w5759, "Device in"=w5761) -> ("error out"=w5755:errorcluster, "Device out"=w5760:refnum<class "Channel.lvclass">)  [unwired: 7 in]
              }
            }
            n2417 = call-dynamic "Write Channel.vi"("error in (no error)"=w5744, "Channel.lvclass"=w5737, "Acquisition in"=w5739) -> ("error out"=w5734:errorcluster, "Acquisition out"=w5733:refnum<class "Acquisition.lvclass">)  [unwired: 7 in]
          }
          frame True {
            # "obs type"
            # "suffix"
            # "object"
            n2418 = call "Read Instrument.lvclass.vi"("S4ACS_GUI in"=w5765) -> ("error out"=w5767:errorcluster, "Instrument.lvclass"=w5769:refnum<class "Instrument.lvclass">, "S4ACS_GUI out"=w5764:refnum<class "S4GUI.lvclass">)  [unwired: 8 in]
            n2419 = call "Read WPROT.vi"("error in (no error)"=w5767, "Instrument in"=w5769) -> ("error out"=w5766:errorcluster, "Opt_Selector.lvclass"=w5768:refnum<class "Opt_Selector.lvclass">)  [unwired: 7 in, 1 out]
            n2420 = call-dynamic "Read sequencia.vi"("error in (no error)"=w5766, "Opt_Selector in"=w5768) -> ("sequencia"=w5763:u16)  [unwired: 7 in, 2 out]
            n2421 = case shown="False" w5771 {
              tunnel: [0 w5831] -> w5770
              tunnel: w5763 -> [_ w5830]
              frame False {
                # "OV 20230424: \n#SEQ agora armazena as\nposições da lâmina utilizadas.\nNa fotometria, #SEQ=0"
                # "fotometria:"
              }
              frame True {
                # "OV 20230424: \n#SEQ agora armazena as\nposições da lâmina utilizadas.\nNa polarimetria, #SEQ=WPROT.sequencia"
                # "polarimetria:"
                n2422 = To Unsigned Long Integer(number=w5830) -> (unsigned 32bit integer=w5831:u32)
              }
            }
            n2423 = call-dynamic "Write Acq_state.vi"("error in (no error)"=w5794, "Acq_state"=u32 251, "Acquisition in"=w5800) -> ("error out"=w5801:errorcluster, "Acquisition out"=w5802:refnum<class "Acquisition.lvclass">)  [unwired: 7 in]
            n2424 = call-dynamic "Read Channel.vi"("error in (no error)"=w5801, "Acquisition in"=w5802) -> ("error out"=w5804:errorcluster, "Channel.lvclass"=w5805:refnum<class "Channel.lvclass">, "Acquisition out"=w5813:refnum<class "Acquisition.lvclass">)  [unwired: 7 in]
            n2425 = property on="Start ch4" class="Bool"(error in=w5794, "DisabledEnum"=T7."Disabled and Grayed Out" ("Disabled")) -> ()  [unwired: 1 in, 2 out]
            n2426 = call-dynamic "Read Interface.vi"("error in (no error)"=w5804, "Channel in"=w5805) -> ("error out"=w5827:errorcluster, "Interface.lvclass"=w5828:refnum<class "Interface.lvclass">, "Channel out"=w5826:refnum<class "Channel.lvclass">)  [unwired: 7 in]
            n2427 = call "Write Exposure Time.vi"("error in (no error)"=w5827, "Exposure Time"="Exptime ch4", "Interface in"=w5828) -> ("error out"=w5824:errorcluster, "Interface out"=w5825:refnum<class "Interface.lvclass">)  [unwired: 7 in]
            n2428 = call-dynamic "Write # Index.vi"("error in (no error)"=w5824, "# Index"="Index ch4", "Interface in"=w5825) -> ("error out"=w5822:errorcluster, "Interface out"=w5823:refnum<class "Interface.lvclass">)  [unwired: 7 in]
            n2429 = call-dynamic "Write Suffix.vi"("error in (no error)"=w5822, "Suffix"=w5796, "Interface in"=w5823) -> ("error out"=w5821:errorcluster, "Interface out"=w5820:refnum<class "Interface.lvclass">)  [unwired: 7 in]
            n2430 = call-dynamic "Write ObsType.vi"("error in (no error)"=w5821, "ObsType"=w5790, "Interface in"=w5820) -> ("error out"=w5818:errorcluster, "Interface out"=w5819:refnum<class "Interface.lvclass">)  [unwired: 7 in]
            n2431 = call-dynamic "Write Object.vi"("error in (no error)"=w5818, "Object"=w5789, "Interface in"=w5819) -> ("error out"=w5817:errorcluster, "Interface out"=w5816:refnum<class "Interface.lvclass">)  [unwired: 7 in]
            n2432 = call-dynamic "Write Comments.vi"("error in (no error)"=w5817, "Comments"=w5795, "Interface in"=w5816) -> ("error out"=w5814:errorcluster, "Interface out"=w5815:refnum<class "Interface.lvclass">)  [unwired: 7 in]
            n2433 = call-dynamic "Write DS9.vi"("error in (no error)"=w5814, "DS9"="F", "Interface in"=w5815) -> ("error out"=w5786:errorcluster, "Interface out"=w5788:refnum<class "Interface.lvclass">)  [unwired: 7 in]
            n2434 = call-dynamic "Write Observer.vi"("error in (no error)"=w5786, "Observer"=w5784, "Interface in"=w5788) -> ("error out"=w5785:errorcluster, "Interface out"=w5787:refnum<class "Interface.lvclass">)  [unwired: 7 in]
            n2435 = call-dynamic "Write # Images.vi"("error in (no error)"=w5785, "# Images"="Exp ch4", "Interface in"=w5787) -> ("error out"=w5791:errorcluster, "Interface out"=w5792:refnum<class "Interface.lvclass">)  [unwired: 7 in]
            n2436 = property on="Exposure Time ch4" class="Slide (strict)"("Scale.Maximum"="Exptime ch4", "Scale.Minimum"=0.0 ("Scale.Range:Minimum")) -> ()  [unwired: 2 in, 2 out]
            n2437 = property on="Exposure Done ch4" class="Slide (strict)"("Scale.Maximum"="Exp ch4", "Scale.Minimum"=0.0 ("Scale.Range:Minimum")) -> ()  [unwired: 2 in, 2 out]
            n2438 = call-dynamic "Write Interface.vi"("error in (no error)"=w5791, "Interface.lvclass"=w5792, "Channel in"=w5826) -> ("error out"=w5806:errorcluster, "Channel out"=w5807:refnum<class "Channel.lvclass">)  [unwired: 7 in]
            n2439 = property on="Cycles Done ch4" class="Slide (strict)"("Scale.Maximum"="#cycles ch4", "Scale.Minimum"=0.0 ("Scale.Range:Minimum")) -> ()  [unwired: 2 in, 2 out]
            n2440 = call-dynamic "Write ciclos.vi"("error in (no error)"=w5806, "ciclos"="#cycles ch4", "Channel in"=w5807) -> ("error out"=w5782:errorcluster, "Channel out"=w5783:refnum<class "Channel.lvclass">)  [unwired: 7 in]
            n2441 = call-dynamic "Write sequencias.vi"("error in (no error)"=w5782, "sequencias"=w5770, "Channel in"=w5783) -> ("error out"=w5781:errorcluster, "Channel out"=w5780:refnum<class "Channel.lvclass">)  [unwired: 7 in]
            n2442 = call-dynamic "Write Channel.vi"("error in (no error)"=w5781, "Channel.lvclass"=w5780, "Acquisition in"=w5813) -> ("error out"=w5774:errorcluster, "Acquisition out"=w5799:refnum<class "Acquisition.lvclass">)  [unwired: 7 in]
            n2443 = call-dynamic "Write sequencias.vi"("error in (no error)"=w5774, "sequencias"=w5770, "S4GUI in"=w5764) -> ("error out"=w5777:errorcluster, "S4GUI out"=w5776:refnum<class "S4GUI.lvclass">)  [unwired: 7 in]
            n2444 = call-dynamic "Write ciclos.vi"("error in (no error)"=w5777, "ciclos"="#cycles ch4", "S4ACS_GUI in"=w5776) -> ("error out"=w5778:errorcluster, "S4ACS_GUI out"=w5779:refnum<class "S4GUI.lvclass">)  [unwired: 7 in]
            n2445 = call-dynamic "Write TotalCiclos.vi"("error in (no error)"=w5778, "TotalCiclos"="#cycles ch4", "S4GUI in"=w5779) -> ("error out"=w5773:errorcluster, "S4GUI out"=w5775:refnum<class "S4GUI.lvclass">)  [unwired: 7 in]
          }
        }
        n2446 = call-dynamic "Write AcquisitionD.vi"("error in (no error)"=w5709, "Acquisition.lvclass"=w5724, "S4ACS_GUI in"=w5708) -> ("error out"=w5723:errorcluster, "S4ACS_GUI out"=w5720:refnum<class "S4GUI.lvclass">)  [unwired: 7 in]
      }
      event "Exptime ch1": Value Change {
        n2447 = event-data() -> ("NewVal"=w5836:dbl)  [unwired: 1 in]
        n2448 = call-dynamic "Read AcquisitionA.vi"("error in (no error)"=w5835, "S4ACS_GUI in"=w5834) -> ("error out"=w5850:errorcluster, "Acquisition.lvclass"=w5851:refnum<class "Acquisition.lvclass">, "S4ACS_GUI out"=w5848:refnum<class "S4GUI.lvclass">)  [unwired: 7 in]
        n2449 = call-dynamic "Read Channel.vi"("error in (no error)"=w5850, "Acquisition in"=w5851) -> ("error out"=w5839:errorcluster, "Channel.lvclass"=w5840:refnum<class "Channel.lvclass">, "Acquisition out"=w5841:refnum<class "Acquisition.lvclass">)  [unwired: 7 in]
        n2450 = call-dynamic "Read Interface.vi"("error in (no error)"=w5839, "Channel in"=w5840) -> ("error out"=w5845:errorcluster, "Interface.lvclass"=w5846:refnum<class "Interface.lvclass">, "Channel out"=w5844:refnum<class "Channel.lvclass">)  [unwired: 7 in]
        n2451 = call "Write Exposure Time.vi"("error in (no error)"=w5845, "Exposure Time"=w5836, "Interface in"=w5846) -> ("error out"=w5837:errorcluster, "Interface out"=w5838:refnum<class "Interface.lvclass">)  [unwired: 7 in]
        n2452 = call-dynamic "Write Interface.vi"("error in (no error)"=w5837, "Interface.lvclass"=w5838, "Channel in"=w5844) -> ("error out"=w5843:errorcluster, "Channel out"=w5842:refnum<class "Channel.lvclass">)  [unwired: 7 in]
        n2453 = call-dynamic "Write Channel.vi"("error in (no error)"=w5843, "Channel.lvclass"=w5842, "Acquisition in"=w5841) -> ("error out"=w5847:errorcluster, "Acquisition out"=w5849:refnum<class "Acquisition.lvclass">)  [unwired: 7 in]
        n2454 = call-dynamic "Write AcquisitionA.vi"("error in (no error)"=w5847, "Acquisition.lvclass"=w5849, "S4ACS_GUI in"=w5848) -> ("error out"=w5833:errorcluster, "S4ACS_GUI out"=w5832:refnum<class "S4GUI.lvclass">)  [unwired: 7 in]
      }
      event "Exp ch1": Value Change {
        n2455 = event-data() -> ("NewVal"=w5856:u32)  [unwired: 1 in]
        n2456 = call-dynamic "Read AcquisitionA.vi"("error in (no error)"=w5855, "S4ACS_GUI in"=w5854) -> ("error out"=w5870:errorcluster, "Acquisition.lvclass"=w5871:refnum<class "Acquisition.lvclass">, "S4ACS_GUI out"=w5868:refnum<class "S4GUI.lvclass">)  [unwired: 7 in]
        n2457 = call-dynamic "Read Channel.vi"("error in (no error)"=w5870, "Acquisition in"=w5871) -> ("error out"=w5859:errorcluster, "Channel.lvclass"=w5860:refnum<class "Channel.lvclass">, "Acquisition out"=w5861:refnum<class "Acquisition.lvclass">)  [unwired: 7 in]
        n2458 = call-dynamic "Read Interface.vi"("error in (no error)"=w5859, "Channel in"=w5860) -> ("error out"=w5865:errorcluster, "Interface.lvclass"=w5866:refnum<class "Interface.lvclass">, "Channel out"=w5864:refnum<class "Channel.lvclass">)  [unwired: 7 in]
        n2459 = call-dynamic "Write Kinetic Series Length.vi"("error in (no error)"=w5865, "Kinetic Series Length"=w5856, "Interface in"=w5866) -> ("error out"=w5857:errorcluster, "Interface out"=w5858:refnum<class "Interface.lvclass">)  [unwired: 7 in]
        n2460 = call-dynamic "Write Interface.vi"("error in (no error)"=w5857, "Interface.lvclass"=w5858, "Channel in"=w5864) -> ("error out"=w5863:errorcluster, "Channel out"=w5862:refnum<class "Channel.lvclass">)  [unwired: 7 in]
        n2461 = call-dynamic "Write Channel.vi"("error in (no error)"=w5863, "Channel.lvclass"=w5862, "Acquisition in"=w5861) -> ("error out"=w5867:errorcluster, "Acquisition out"=w5869:refnum<class "Acquisition.lvclass">)  [unwired: 7 in]
        n2462 = call-dynamic "Write AcquisitionA.vi"("error in (no error)"=w5867, "Acquisition.lvclass"=w5869, "S4ACS_GUI in"=w5868) -> ("error out"=w5853:errorcluster, "S4ACS_GUI out"=w5852:refnum<class "S4GUI.lvclass">)  [unwired: 7 in]
      }
      event "Stop ch1": Value Change {
        n2463 = event-data() -> ()  [unwired: 1 in, 6 out]
        n2464 = disable-structure shown="Enabled" {
          disable-tunnel: w5875 -> [w5908 w5936]
          disable-tunnel: w5874 -> [w5906 w5929]
          disable-tunnel: [w5888 w5928] -> w5873
          disable-tunnel: [w5876 w5936] -> w5872
          frame Disabled {
            # "Para movimento \nda lamina retardadora"
            # "Restaura a última sequência de lâminas"
            n2465 = call-dynamic "Read AcquisitionA.vi"("error in (no error)"=w5906, "S4ACS_GUI in"=w5908) -> ("error out"=w5910:errorcluster, "Acquisition.lvclass"=w5909:refnum<class "Acquisition.lvclass">, "S4ACS_GUI out"=w5907:refnum<class "S4GUI.lvclass">)  [unwired: 7 in]
            n2466 = disable-structure shown="Enabled" {
              disable-tunnel: w5910 -> [w5915 w5926]
              disable-tunnel: w5909 -> [w5914 w5927]
              disable-tunnel: [w5912 w5927] -> w5904
              disable-tunnel: [w5911 w5926] -> w5903
              frame Disabled {
                # "Só precisa enviar comando STOP quando\no controle dos ciclos for feito pelo ACS."
                n2467 = call-dynamic "Read Channel.vi"("error in (no error)"=w5915, "Acquisition in"=w5914) -> ("error out"=w5917:errorcluster, "Channel.lvclass"=w5916:refnum<class "Channel.lvclass">, "Acquisition out"=w5923:refnum<class "Acquisition.lvclass">)  [unwired: 7 in]
                n2468 = call-dynamic "Read State Machine.vi"("error in (no error)"=w5917, "Device in"=w5916) -> ("error out"=w5919:errorcluster, "State Machine.lvclass"=w5918:refnum<class "State Machine.lvclass">, "Device out"=w5921:refnum<class "Channel.lvclass">)  [unwired: 7 in]
                n2469 = call "Next State.vi"("error in (no error)"=w5919, "New_State"=u32 70, "State Machine in"=w5918) -> ("error out"=w5922:errorcluster, "State Machine out"=w5920:refnum<class "State Machine.lvclass">)  [unwired: 7 in]
                n2470 = call-dynamic "Write State Machine.vi"("error in (no error)"=w5922, "State Machine.lvclass"=w5920, "Device in"=w5921) -> ("error out"=w5924:errorcluster, "Device out"=w5925:refnum<class "Channel.lvclass">)  [unwired: 7 in]
                n2471 = call-dynamic "Write Channel.vi"("error in (no error)"=w5924, "Channel.lvclass"=w5925, "Acquisition in"=w5923) -> ("error out"=w5911:errorcluster, "Acquisition out"=w5912:refnum<class "Acquisition.lvclass">)  [unwired: 7 in]
              }
              frame Enabled {
                # "Não precisa enviar comando STOP para o ACS\nenquanto o controle dos ciclos for feito pela GUI."
              }
            }
            n2472 = call-dynamic "Write Acq_state.vi"("error in (no error)"=w5903, "Acq_state"=u32 0, "Acquisition in"=w5904) -> ("error out"=w5902:errorcluster, "Acquisition out"=w5901:refnum<class "Acquisition.lvclass">)  [unwired: 7 in]
            n2473 = call-dynamic "Write AcquisitionA.vi"("error in (no error)"=w5902, "Acquisition.lvclass"=w5901, "S4ACS_GUI in"=w5907) -> ("error out"=w5889:errorcluster, "S4ACS_GUI out"=w5887:refnum<class "S4GUI.lvclass">)  [unwired: 7 in]
            n2474 = call "Read Instrument.lvclass.vi"("error in (no error)"=w5889, "S4ACS_GUI in"=w5887) -> ("error out"=w5896:errorcluster, "Instrument.lvclass"=w5899:refnum<class "Instrument.lvclass">, "S4ACS_GUI out"=w5900:refnum<class "S4GUI.lvclass">)  [unwired: 7 in]
